vi "MagnetQuery.vi"(9 "VISA resource name":refnum<visa-resource-name>="TCPIP0::192.168.128.3::7020::SOCKET") -> (0 "Set Field (T)":dbl, 1 "Helium Level (%)":dbl, 2 "Field from current in leads (T)":dbl, 3 "Real Field (T)":dbl, 4 "STATUS":string, 5 "Status Buttons":enum32{"HOLD", "To Set", "To Zero", "To Zero 2"}(radio), 6 "Switch Heater Status":string, 7 "Switch Heater":bool)   [LabVIEW 2015]
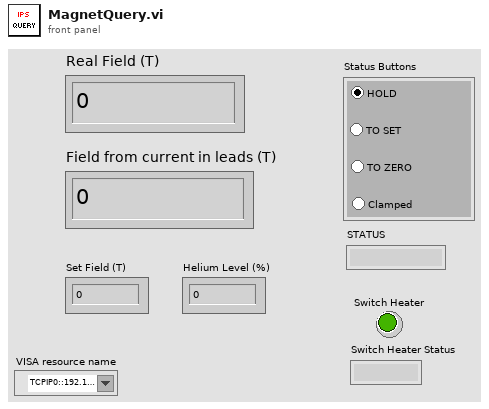
[diagram p1: front panel]
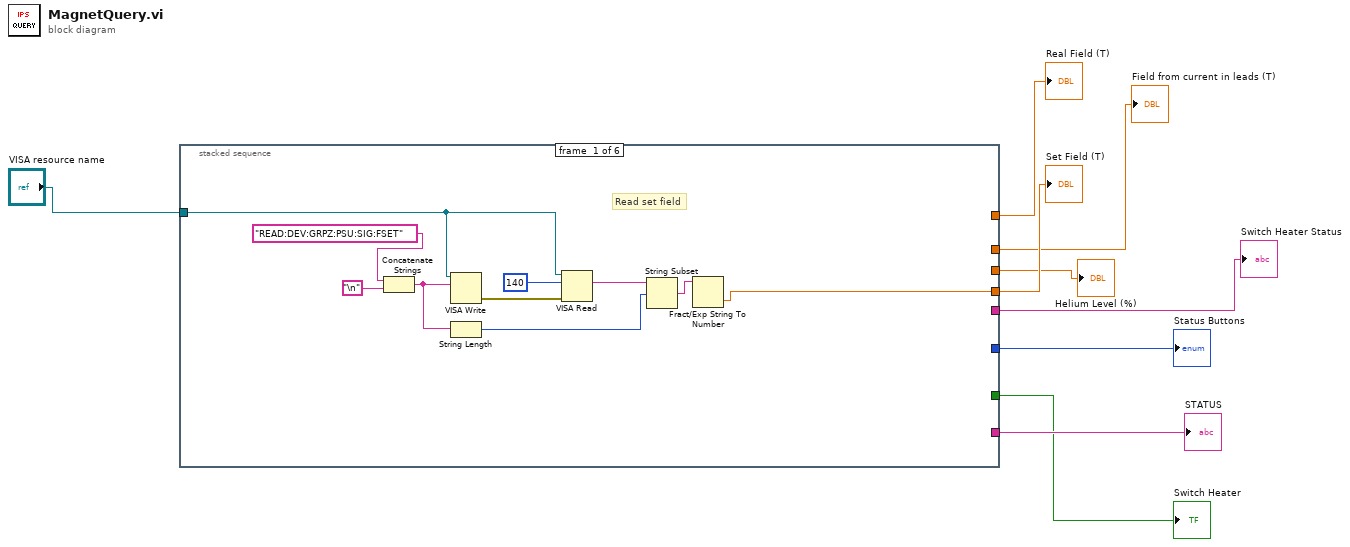
[diagram p0: block diagram]
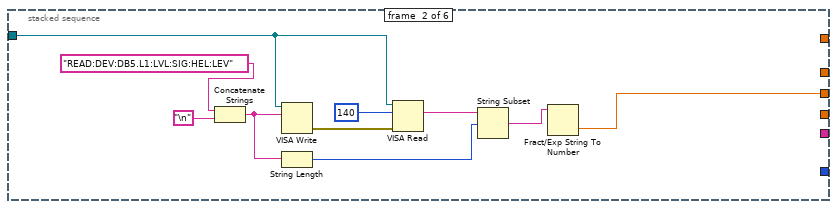
[diagram p2: hidden frame]
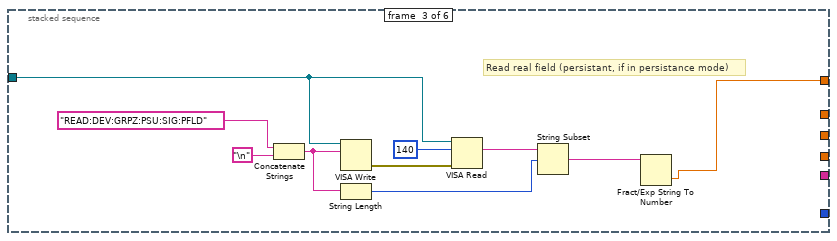
[diagram p3: hidden frame]
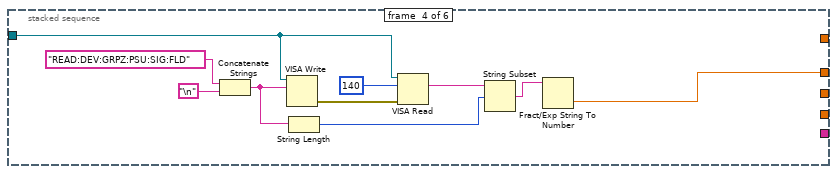
[diagram p4: hidden frame]
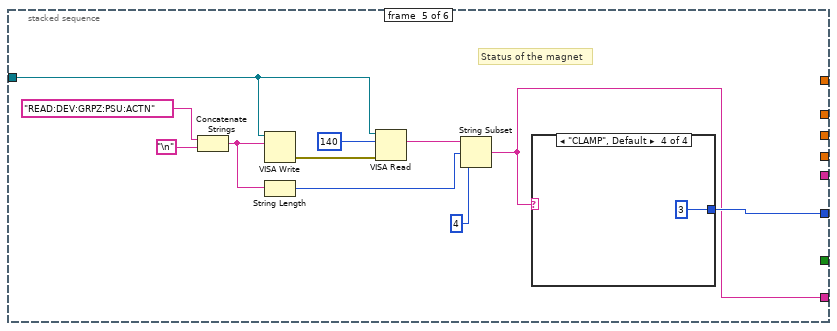
[diagram p5: hidden frame]
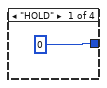
[diagram p6: hidden frame]
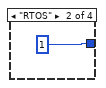
[diagram p7: hidden frame]
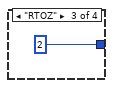
[diagram p8: hidden frame]
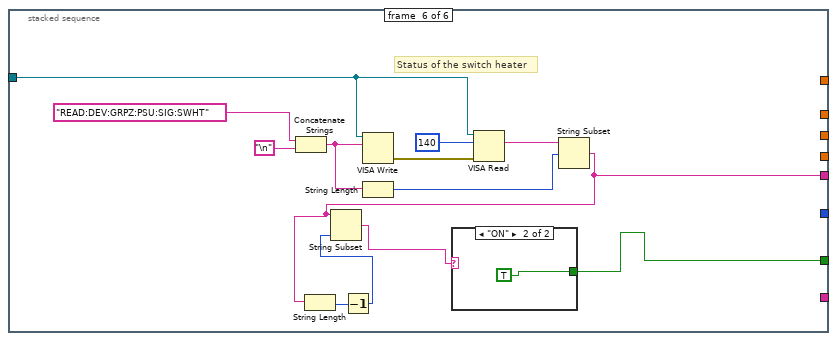
[diagram p9: hidden frame]
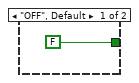
[diagram p10: hidden frame]
diagram:
  n1 = stacked-sequence {
    tunnel: "VISA resource name" -> [w11 w21 w31 w41 w53 w70]
    tunnel: [w10 _ _ _ _ _] -> w8
    tunnel: [_ w20 _ _ _ _] -> w7
    tunnel: [_ _ w30 _ _ _] -> w6
    tunnel: [_ _ _ w40 _ _] -> w5
    tunnel: [_ _ _ _ w51 _] -> w4
    tunnel: [_ _ _ _ w50 _] -> w3
    tunnel: [_ _ _ _ _ w66] -> w2
    tunnel: [_ _ _ _ _ w65] -> w1
    frame #0 {
      # "Read set field"
      n2 = Concatenate Strings("READ:DEV:GRPZ:PSU:SIG:FSET" ("string"), "\n") -> (w13:string)
      n3 = VISA Write(VISA resource name=w11, write buffer=w13) -> (error out=w19:errorcluster)  [unwired: 1 in, 2 out]
      n4 = String Length(string=w13) -> (length=w14:i32)
      n5 = VISA Read(VISA resource name=w11, byte count=140, error in (no error)=w19) -> (read buffer=w15:string)  [unwired: 3 out]
      n6 = String Subset(string=w15, offset (0)=w14) -> (substring=w12:string)  [unwired: 1 in]
      n7 = Fract/Exp String To Number(string=w12) -> (number=w10:dbl)  [unwired: 3 in, 1 out]
    }
    frame #1 {
      n8 = Concatenate Strings("READ:DEV:DB5.L1:LVL:SIG:HEL:LEV" ("string"), "\n") -> (w23:string)
      n9 = VISA Write(VISA resource name=w21, write buffer=w23) -> (error out=w29:errorcluster)  [unwired: 1 in, 2 out]
      n10 = String Length(string=w23) -> (length=w24:i32)
      n11 = VISA Read(VISA resource name=w21, byte count=140, error in (no error)=w29) -> (read buffer=w25:string)  [unwired: 3 out]
      n12 = String Subset(string=w25, offset (0)=w24) -> (substring=w22:string)  [unwired: 1 in]
      n13 = Fract/Exp String To Number(string=w22) -> (number=w20:dbl)  [unwired: 3 in, 1 out]
    }
    frame #2 {
      # "Read real field (persistant, if in persistance mode)"
      n14 = Concatenate Strings("READ:DEV:GRPZ:PSU:SIG:PFLD" ("string"), "\n") -> (w33:string)
      n15 = VISA Write(VISA resource name=w31, write buffer=w33) -> (error out=w39:errorcluster)  [unwired: 1 in, 2 out]
      n16 = String Length(string=w33) -> (length=w34:i32)
      n17 = VISA Read(VISA resource name=w31, byte count=140, error in (no error)=w39) -> (read buffer=w35:string)  [unwired: 3 out]
      n18 = String Subset(string=w35, offset (0)=w34) -> (substring=w32:string)  [unwired: 1 in]
      n19 = Fract/Exp String To Number(string=w32) -> (number=w30:dbl)  [unwired: 3 in, 1 out]
    }
    frame #3 {
      n20 = Concatenate Strings("READ:DEV:GRPZ:PSU:SIG:FLD" ("string"), "\n") -> (w45:string)
      n21 = VISA Write(VISA resource name=w41, write buffer=w45) -> (error out=w49:errorcluster)  [unwired: 1 in, 2 out]
      n22 = String Length(string=w45) -> (length=w43:i32)
      n23 = VISA Read(VISA resource name=w41, byte count=140, error in (no error)=w49) -> (read buffer=w44:string)  [unwired: 3 out]
      n24 = String Subset(string=w44, offset (0)=w43) -> (substring=w42:string)  [unwired: 1 in]
      n25 = Fract/Exp String To Number(string=w42) -> (number=w40:dbl)  [unwired: 3 in, 1 out]
    }
    frame #4 {
      # "Status of the magnet"
      n26 = Concatenate Strings("READ:DEV:GRPZ:PSU:ACTN" ("string"), "\n") -> (w54:string)
      n27 = VISA Write(VISA resource name=w53, write buffer=w54) -> (error out=w60:errorcluster)  [unwired: 1 in, 2 out]
      n28 = String Length(string=w54) -> (length=w55:i32)
      n29 = VISA Read(VISA resource name=w53, byte count=140, error in (no error)=w60) -> (read buffer=w56:string)  [unwired: 3 out]
      n30 = String Subset(string=w56, offset (0)=w55, length (rest)=4) -> (substring=w50:string)
      n31 = case shown="\"CLAMP\", Default" w50 {
        tunnel: [0 1 2 3] -> w51
        frame "HOLD" {
        }
        frame "RTOS" {
        }
        frame "RTOZ" {
        }
        frame "CLAMP", Default {
        }
      }
    }
    frame #5 {
      # "Status of the switch heater"
      n32 = Concatenate Strings("READ:DEV:GRPZ:PSU:SIG:SWHT" ("string"), "\n") -> (w71:string)
      n33 = VISA Write(VISA resource name=w70, write buffer=w71) -> (error out=w77:errorcluster)  [unwired: 1 in, 2 out]
      n34 = String Length(string=w71) -> (length=w72:i32)
      n35 = VISA Read(VISA resource name=w70, byte count=140, error in (no error)=w77) -> (read buffer=w73:string)  [unwired: 3 out]
      n36 = String Subset(string=w73, offset (0)=w72) -> (substring=w66:string)  [unwired: 1 in]
      n37 = String Length(string=w66) -> (length=w69:i32)
      n38 = Decrement(x=w69) -> (x-1=w68:i32)
      n39 = String Subset(string=w66, length (rest)=w68) -> (substring=w67:string)  [unwired: 1 in]
      n40 = case shown="\"ON\"" w67 {
        tunnel: [FALSE TRUE] -> w65
        frame "OFF", Default {
        }
        frame "ON" {
        }
      }
    }
  }
  "Set Field (T)" <- w8
  "Helium Level (%)" <- w7
  "Real Field (T)" <- w6
  "Field from current in leads (T)" <- w5
  "Status Buttons" <- w4
  "STATUS" <- w3
  "Switch Heater Status" <- w2
  "Switch Heater" <- w1
